vi "DS18x20 - top level.vi"(6 "Reset Delay (ms)":u32=100, 7 "1-Wire DIO Pin":refnum<k21>="ConnectorA/DIO15", 8 "error in":errorcluster, 9 "Master Function Command":T1, 10 "ROM Command":T2=enum."Skip ROM Command") -> (0 "error out":errorcluster, 1 "Scratchpad Data":u8[](array[numeric]) format="%.0x", 2 "ROM Data":u8[](array[numeric]) format="%.0x", 4 "Convert Time (usec)":u32, 5 "Supply Mode":bool)   [LabVIEW 2014]
uses:
  ROM Commands.ctl
  Master Function Commands.ctl
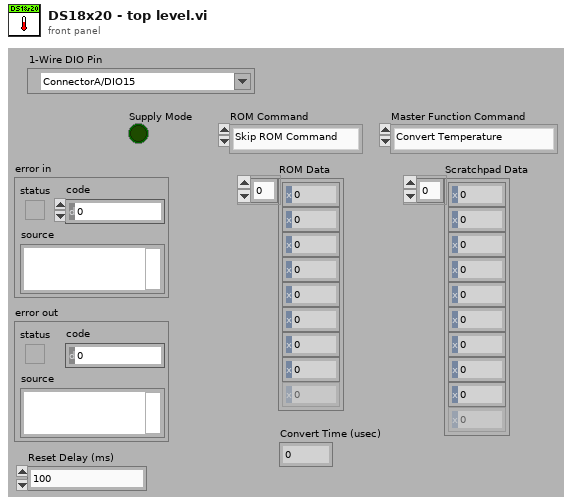
[diagram p1: front panel]
types:
  T1 = typedef "Master Function Commands.ctl" = enum16{"Convert Temperature", "Read Scratchpad", "Read Power Supply"}
  T2 = typedef "ROM Commands.ctl" = enum16{"Read ROM", "Skip ROM Command"}
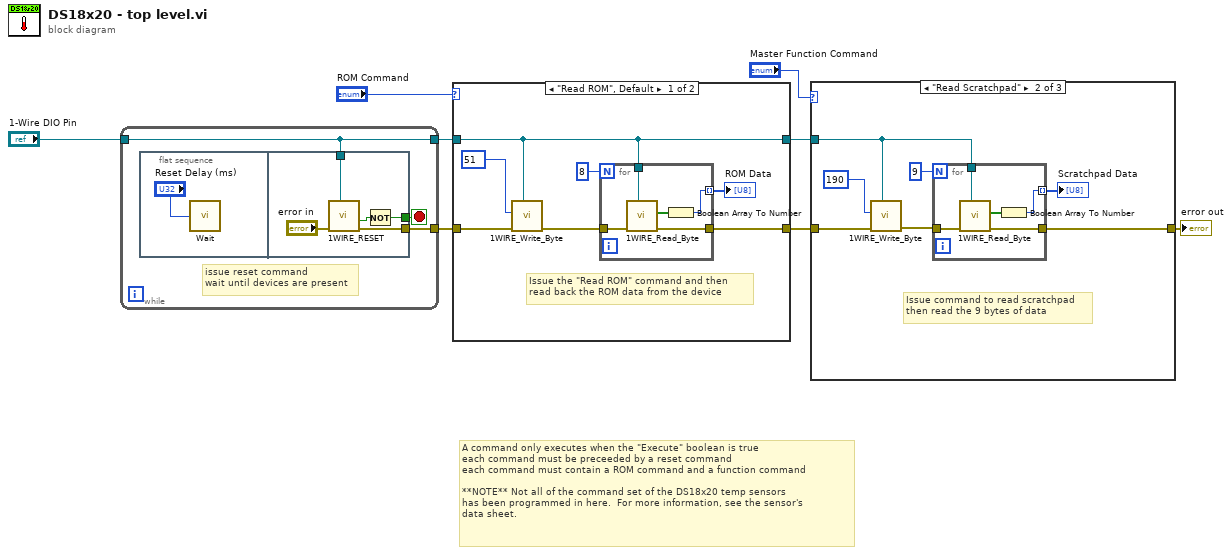
[diagram p0: block diagram]
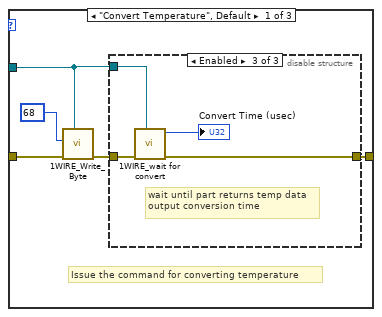
[diagram p2: hidden frame]
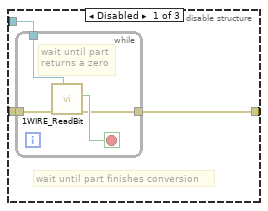
[diagram p3: hidden frame]
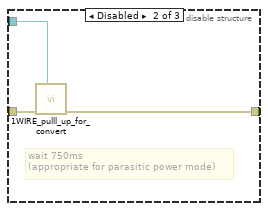
[diagram p4: hidden frame]
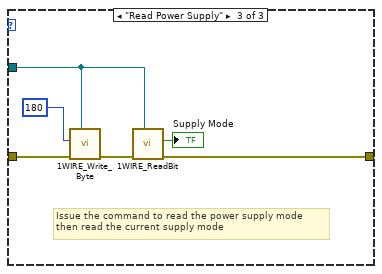
[diagram p5: hidden frame]
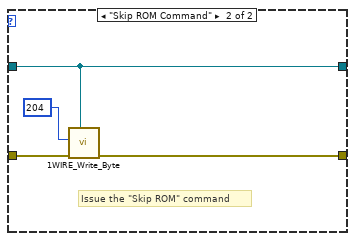
[diagram p6: hidden frame]
diagram:
  # "A command only executes when the \"Execute\" boolean is true\neach command must be preceeded by a reset command\neach command must contain a ROM command and a function command\n\n**NOTE** Not all of the command set of the DS18x20 temp sensors\nhas been programmed in here.  For more information, see the sensor's\ndata sheet."
  n1 = while {
    tunnel: [w10] -> w5
    tunnel: "1-Wire DIO Pin" -> [w9]
    tunnel: [w9] -> w2
    stop <- w11 stop-if-true
    # "issue reset command\nwait until devices are present"
    n2 = flat-sequence {
      tunnel: [w16] -> w11
      tunnel: [w15] -> w10
      tunnel: w9 -> [w13]
      frame #0 {
        n3 = call "Wait"("Count(mSec)"="Reset Delay (ms)") -> ()  [unwired: 1 out]
      }
      frame #1 {
        n4 = call "1WIRE_RESET.vi"("1-Wire DIO Pin"=w13, "error in"="error in") -> ("error out"=w15:errorcluster, "0 = Device Present / 1=no"=w14:bool)  [unwired: 8 in]
        n5 = Not(x=w14) -> (.not. x?=w16:bool)
      }
    }
  }
  n6 = case shown="\"Read ROM\", Default" "ROM Command" {
    tunnel: w5 -> [w22 w33]
    tunnel: [w20 w32] -> w4
    tunnel: w2 -> [w18 w30]
    tunnel: [w18 w30] -> w1
    frame "Read ROM", Default {
      # "Issue the \"Read ROM\" command and then\nread back the ROM data from the device"
      n7 = call "1WIRE_Write_Byte.vi"("1-Wire DIO Pin"=w18, "error in"=w22, "Tx data"=u8 51 ("Tx data 2")) -> ("error out"=w24:errorcluster)  [unwired: 7 in, 1 out]
      n8 = for {
        N: 8 -> [_]
        tunnel: w24 -> [w29]
        tunnel: [w28] -> w20
        tunnel: [w26] -> w21 mode=indexing
        tunnel: w18 -> [w25]
        n9 = call "1WIRE_Read_Byte.vi"("1-Wire DIO Pin"=w25, "error in"=w29) -> ("error out"=w28:errorcluster, "Array"=w27:bool[])  [unwired: 8 in]
        n10 = Boolean Array To Number(Boolean array=w27) -> (number=w26:u8)
      }
      "ROM Data" <- w21
    }
    frame "Skip ROM Command" {
      # "Issue the \"Skip ROM\" command"
      n11 = call "1WIRE_Write_Byte.vi"("1-Wire DIO Pin"=w30, "error in"=w33, "Tx data"=u8 204) -> ("error out"=w32:errorcluster)  [unwired: 7 in, 1 out]
    }
  }
  n12 = case shown="\"Read Scratchpad\"" "Master Function Command" {
    tunnel: w4 -> [w38 w56 w69]
    tunnel: [w36 w55 w67] -> w6
    tunnel: w1 -> [w34 w53 w65]
    frame "Convert Temperature", Default {
      # "Issue the command for converting temperature"
      n13 = call "1WIRE_Write_Byte.vi"("1-Wire DIO Pin"=w34, "error in"=w38, "Tx data"=u8 68 ("Tx data 2")) -> ("error out"=w37:errorcluster)  [unwired: 7 in, 1 out]
      n14 = disable-structure shown="Enabled" {
        disable-tunnel: w37 -> [w41 w48 w52]
        disable-tunnel: [w40 w47 w51] -> w36
        disable-tunnel: w34 -> [w39 w46 w49]
        frame Disabled {
          # "wait until part finishes conversion"
          n15 = while {
            tunnel: w41 -> [w45]
            tunnel: [w43] -> w40
            tunnel: w39 -> [w42]
            stop <- w44 stop-if-true
            # "wait until part\nreturns a zero"
            n16 = call "1WIRE_ReadBit.vi"("1-Wire DIO Pin"=w42, "error in"=w45) -> ("error out"=w43:errorcluster, "Bit Read"=w44:bool)  [unwired: 8 in]
          }
        }
        frame Disabled {
          # "wait 750ms\n(appropriate for parasitic power mode)"
          n17 = call "1WIRE_pulll_up_for_convert.vi"("1-Wire DIO Pin"=w46, "error in"=w48) -> ("error out"=w47:errorcluster)  [unwired: 9 in]
        }
        frame Enabled {
          # "wait until part returns temp data\noutput conversion time"
          n18 = call "1WIRE_wait for convert.vi"("1-Wire DIO Pin"=w49, "error in"=w52) -> ("error out"=w51:errorcluster, "Convert Time (usec)"=→"Convert Time (usec)":u32)  [unwired: 8 in]
        }
      }
    }
    frame "Read Scratchpad" {
      # "Issue command to read scratchpad\nthen read the 9 bytes of data"
      n19 = call "1WIRE_Write_Byte.vi"("1-Wire DIO Pin"=w53, "error in"=w56, "Tx data"=u8 190 ("Tx data 2")) -> ("error out"=w57:errorcluster)  [unwired: 7 in, 1 out]
      n20 = for {
        N: 9 -> [_]
        tunnel: w57 -> [w64]
        tunnel: [w63] -> w55
        tunnel: [w61] -> w59 mode=indexing
        tunnel: w53 -> [w60]
        n21 = call "1WIRE_Read_Byte.vi"("1-Wire DIO Pin"=w60, "error in"=w64) -> ("error out"=w63:errorcluster, "Array"=w62:bool[])  [unwired: 8 in]
        n22 = Boolean Array To Number(Boolean array=w62) -> (number=w61:u8)
      }
      "Scratchpad Data" <- w59
    }
    frame "Read Power Supply" {
      # "Issue the command to read the power supply mode\nthen read the current supply mode"
      n23 = call "1WIRE_Write_Byte.vi"("1-Wire DIO Pin"=w65, "error in"=w69, "Tx data"=u8 180 ("Tx data 2")) -> ("error out"=w68:errorcluster)  [unwired: 7 in, 1 out]
      n24 = call "1WIRE_ReadBit.vi"("1-Wire DIO Pin"=w65, "error in"=w68) -> ("error out"=w67:errorcluster, "Bit Read"=→"Supply Mode":bool)  [unwired: 8 in]
    }
  }
  "error out" <- w6
